vi "AutoCHOPChippyChipChopChopperTopLopper.vi"(9 "Points to chop off the bottom edge":i32, 10 "Points to chop off the top edge":i32, 11 "Vsrc and Current In":cluster{dbl[], dbl[]}) -> (3 "Vsrc and Current Out":cluster{dbl[], dbl[]})   [LabVIEW 2016]
panel:
  in  "zeroes to chop off":i32=205
  out "min index(es)":i32
  out "max index(es)":i32
  out "Entire Current":dbl[](graph)
  out "Entire Vsrc":dbl[](graph)
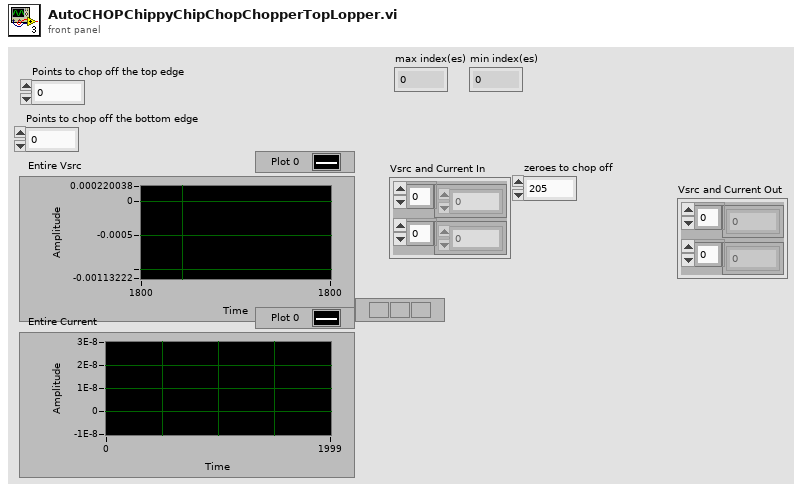
[diagram p1: front panel]
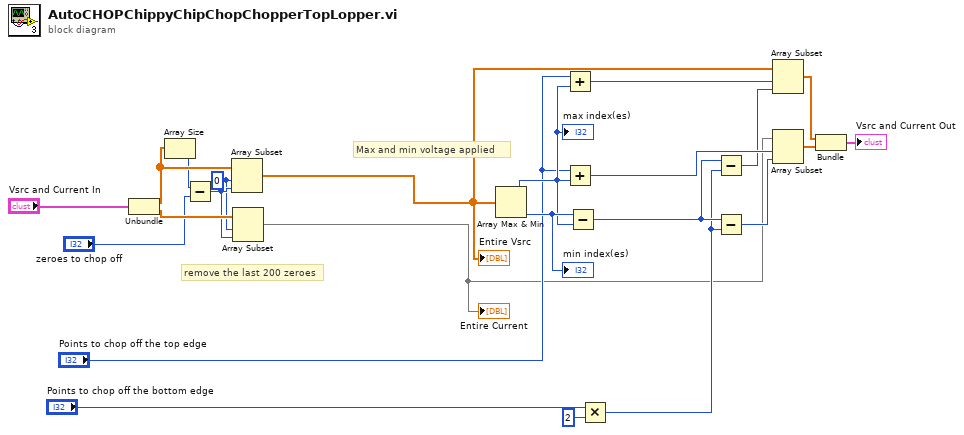
[diagram p0: block diagram]
diagram:
  w3 = 0 ("index")
  # "remove the last 200 zeroes"
  # "Max and min voltage applied"
  n1 = Unbundle("Vsrc and Current In") -> (w7:dbl[], w8:dbl[])
  n2 = Array Size(array=w7) -> (size(s)=w6:i32)
  n3 = Subtract(x=w6, y="zeroes to chop off") -> (x-y=w4:i32)
  n4 = Array Subset(array=w7, index=w3, length=w4) -> (w2:dbl[])
  "Entire Vsrc" <- w2
  n5 = Array Subset(array=w8, index=w3, length=w4) -> (w1:dbl[])
  "Entire Current" <- w1
  n6 = Array Max & Min(array=w2) -> (max index (indices)=w18:i32, min index (indices)=w23:i32)  [unwired: 2 out]
  "max index(es)" <- w18
  "min index(es)" <- w23
  n7 = Add(x="Points to chop off the top edge", y=w18) -> (x+y=w22:i32)
  n8 = Add(x="Points to chop off the top edge", y=w18) -> (x+y=w21:i32)
  n9 = Subtract(x=w23, y=w18) -> (x-y=w17:i32)
  n10 = Multiply(x="Points to chop off the bottom edge", y=2) -> (x*y=w13:i32)
  n11 = Subtract(x=w17, y=w13) -> (x-y=w20:i32)
  n12 = Subtract(x=w17, y=w13) -> (x-y=w19:i32)
  n13 = Array Subset(array=w2, index=w22, length=w20) -> (w12:dbl[])
  n14 = Array Subset(array=w1, index=w21, length=w19) -> (w11:dbl[])
  n15 = Bundle(w12, w11) -> (→"Vsrc and Current Out":cluster{dbl[], dbl[]})  [unwired: 1 in]
